vi "AG-UC2-UC8_Close.vi"(3 "error in (no error)":errorcluster caption="error in", 5 "AG-UC2-UC8 Reference":refnum<k24>) -> (0 "Error out":errorcluster caption="error out", 1 "Error":i32)   [LabVIEW 2016]
uses:
  C:/Program Files/Newport/Piezo Motion Control/Newport AG-UC2-UC8 Applet/Samples/LabVIEW 2009/AgilisCmdLib.dll
  Program Files/Newport/Piezo Motion Control/Newport AG-UC2-UC8 Applet/Samples/LabVIEW 2009/AgilisCmdLib.dll
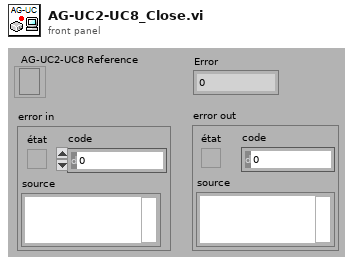
[diagram p1: front panel]
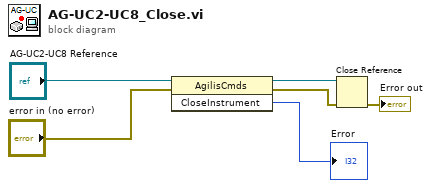
[diagram p0: block diagram]
diagram:
  n1 = invoke class="AgilisCmds" method="CloseInstrument"(reference="AG-UC2-UC8 Reference", error in="error in (no error)") -> (reference out=w6:refnum<k24>, error out=w5:errorcluster, "CloseInstrument"=→"Error":i32)  [unwired: 1 in]
  n2 = Close Reference(reference=w6, error in (no error)=w5) -> (error out=→"Error out":errorcluster)
